vi "Open VI by Test Name.vi"(8 "error in (no error)":errorcluster, 11 "Tag":string) -> (0 "error in (no error) 2":errorcluster)   [LabVIEW 2020, in "Execution UI.lvclass"]
uses:
  Execution UI.lvclass
  Execution UI.lvclass/Execution UI.ctl
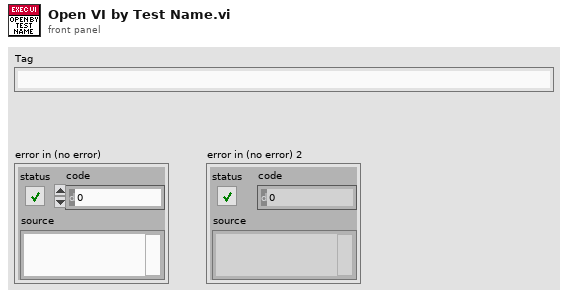
[diagram p1: front panel]
types:
  T1 = enum32{"Invalid", "Standard", "Closed", "Hidden", "Minimized", "Maximized"}
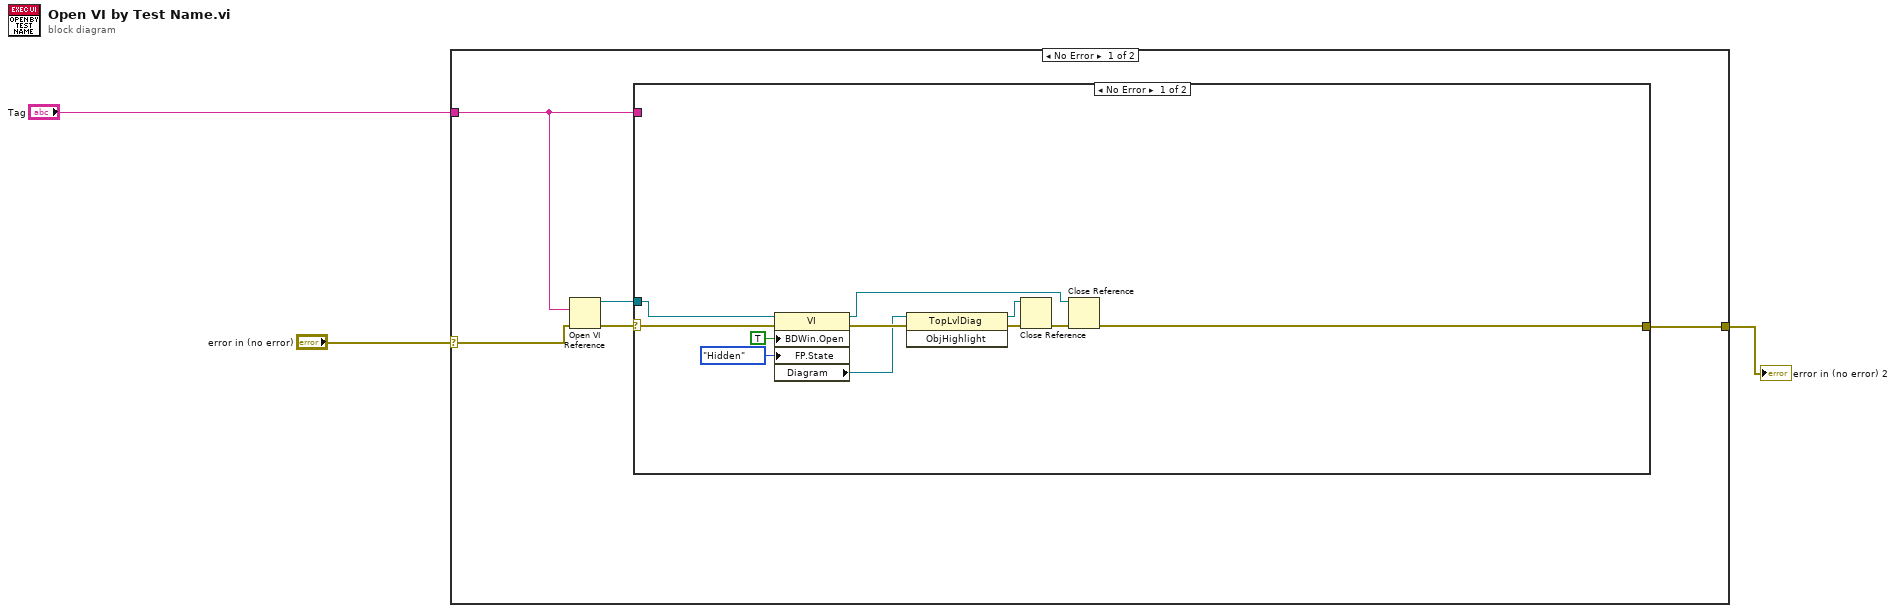
[diagram p0: block diagram]
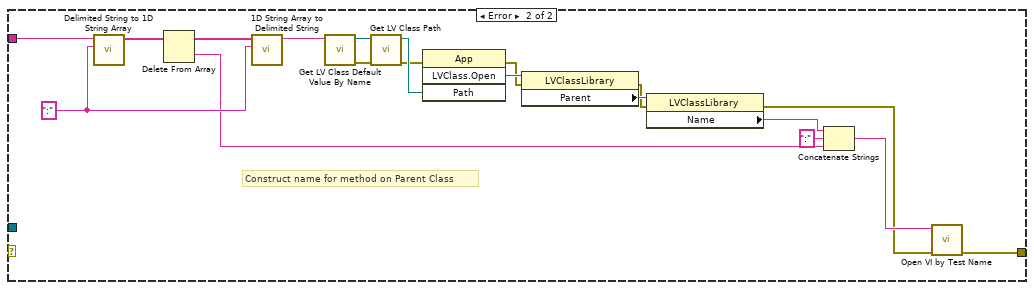
[diagram p2: hidden frame]
diagram:
  n1 = case shown="No Error" "error in (no error)" {
    selector: "error in (no error)" -> [w5 w39]
    tunnel: "Tag" -> [w6 _]
    tunnel: [w4 w39] -> w1
    frame No Error {
      n2 = Open VI Reference(vi path=w6, error in (no error)=w5) -> (vi reference=w8:refnum<vi>, error out=w7:errorcluster)  [unwired: 4 in]
      n3 = case shown="No Error" w7 {
        selector: w7 -> [w14 _]
        tunnel: w8 -> [w16 _]
        tunnel: w6 -> [_ w35]
        tunnel: [w19 w24] -> w4
        frame No Error {
          n4 = property class="VI"(reference=w16, error in=w14, "BDWin.Open"=TRUE ("Block Diagram Window:Open"), "FP.State"=T1."Hidden" ("Front Panel Window:State")) -> (reference out=w17:refnum<vi>, error out=w15:errorcluster, "Diagram"=w11:refnum<vi>)
          n5 = invoke class="TopLvlDiag" method="ObjHighlight"(reference=w11, error in=w15) -> (reference out=w9:refnum<vi>, error out=w12:errorcluster)  [unwired: 1 in, 1 out]
          n6 = Close Reference(reference=w9, error in (no error)=w12) -> (error out=w10:errorcluster)
          n7 = Close Reference(reference=w17, error in (no error)=w10) -> (error out=w19:errorcluster)
        }
        frame Error {
          w36 = ":" ("delimiter")
          # "Construct name for method on Parent Class"
          n8 = call <vilib>:"Delimited String to 1D String Array.vi"("delimiter"=w36, "delimited string"=w35) -> ("string array"=w37:string[])  [unwired: 9 in]
          n9 = Delete From Array(array=w37) -> (deleted portion=w26:string, array with subset deleted=w38:string[])  [unwired: 2 in]
          n10 = call <vilib>:"1D String Array to Delimited String.vi"("delimiter"=w36, "string array"=w38) -> ("delimited string"=w34:string)  [unwired: 9 in]
          n11 = call <vilib>:"Get LV Class Default Value By Name.vi"("class name"=w34) -> ("error out"=w33:errorcluster, "object"=w32:refnum<class>)  [unwired: 9 in]
          n12 = call <vilib>:"Get LV Class Path.vi"("error in (no error)"=w33, "object"=w32) -> ("error out"=w30:errorcluster, "class path"=w31:path)  [unwired: 8 in]
          n13 = invoke class="App" method="LVClass.Open"(error in=w30, "Path"=w31) -> (error out=w21:errorcluster, "LVClass.Open"=w29:refnum<vi>)  [unwired: 2 in, 2 out]
          n14 = property class="LVClassLibrary"(reference=w29, error in=w21) -> (error out=w22:errorcluster, "Parent"=w28:refnum<vi>)  [unwired: 1 out]
          n15 = property class="LVClassLibrary"(reference=w28, error in=w22) -> (error out=w23:errorcluster, "Name"=w27:string)  [unwired: 1 out]
          n16 = Concatenate Strings(w27, ":" ("string"), w26) -> (w25:string)
          n17 = call "Open VI by Test Name.vi"("error in (no error)"=w23, "Tag"=w25) -> ("error in (no error) 2"=w24:errorcluster)  [unwired: 9 in]
        }
      }
    }
    frame Error {
    }
  }
  "error in (no error) 2" <- w1
